vi "FlowCalculation.vi"(6 "order":i32=2, 9 "lowpass":dbl=1.0, 10 "Filter":u16(ring)=2 items=["IIR", "Butterworth", "None"], 11 "X":dbl[](array[numeric]) format="%0.2f") -> (0 "Max amplitude":dbl, 1 "Descending":dbl, 2 "Ascending":dbl, 3 "Flow Graph":T2(graph), 4 "Slopes Out":T1)   [LabVIEW 2013, in "main.lvlib"]
uses:
  main.lvlib
  <vilib>/Analysis/3filter.llb/Filter Passband Type.ctl
  <vilib>/Analysis/3filter.llb/IIR Filter (DBL).vi
  <vilib>/Analysis/3filter.llb/Butterworth Filter (DBL).vi
  <vilib>/Analysis/NI_AALPro.lvlib
  <vilib>/Analysis/NI_AALBase.lvlib
  <vilib>/Analysis/NI_AAL_SigProc.lvlib
panel:
  out "Raw":dbl[](graph)
  out "Derivative Signal":dbl[](graph)
  out "Input Signal":dbl[](graph)
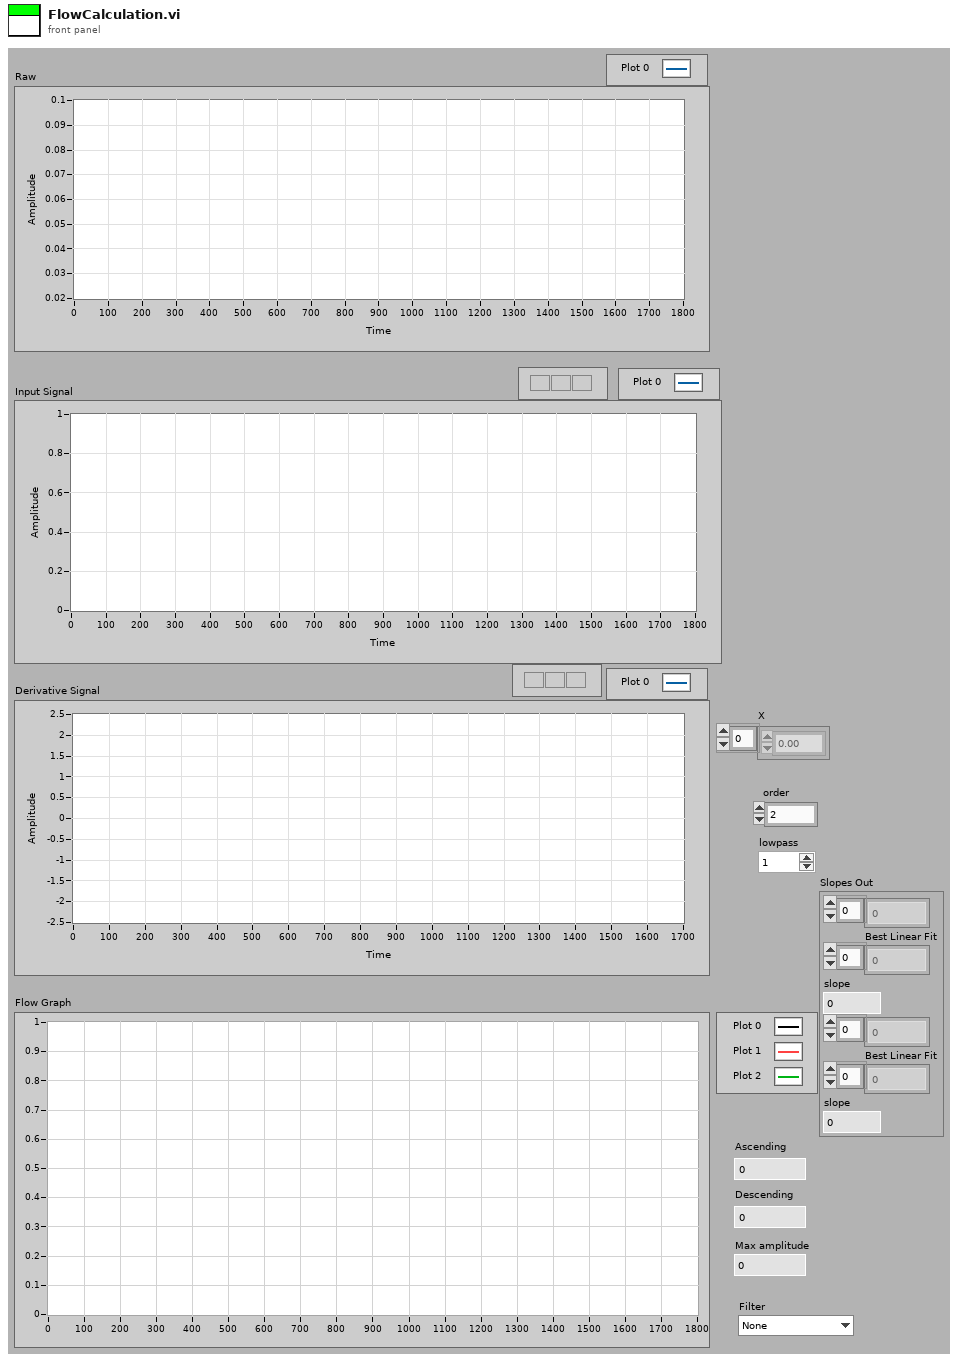
[diagram p1: front panel]
types:
  T1 = cluster{dbl[], "Best Linear Fit":dbl[], "slope":dbl, dbl[], "Best Linear Fit":dbl[], "slope":dbl}
  T2 = cluster{"Array out":dbl[], "Best Linear Fit":dbl[]}[]
  T3 = typedef "NI_AALBase.lvlib/Filter Passband Type.ctl" = enum32{"Lowpass", "Highpass", "Bandpass", "Bandstop"}
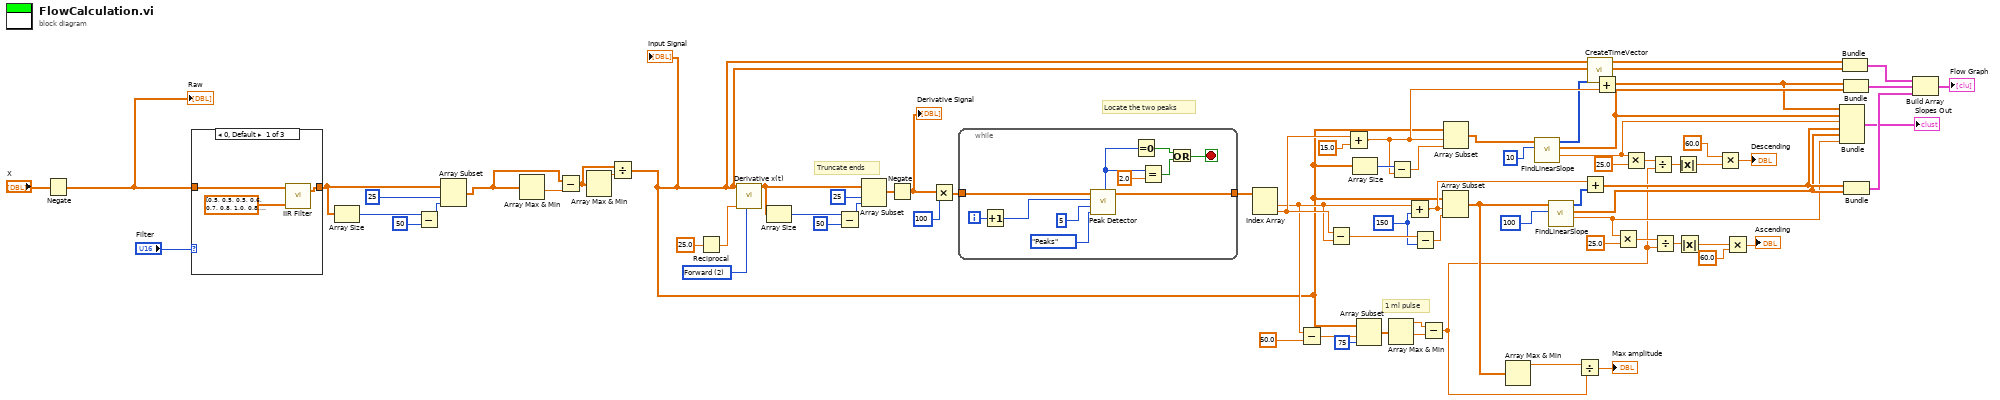
[diagram p0: block diagram]
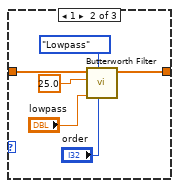
[diagram p2: hidden frame]
diagram:
  w37 = 150
  w75 = u16 2 items=["2nd Order Central", "4th Order Central", "Forward", "Backward"] ("method")
  # "1 ml pulse"
  # "Truncate ends"
  # "Locate the two peaks"
  n1 = Negate(x="X") -> (-x=w19:dbl[])
  "Raw" <- w19
  n2 = case shown="0, Default" "Filter" {
    tunnel: w19 -> [w78 w84 w85]
    tunnel: [w77 w81 w85] -> w12
    frame 0, Default {
      n3 = call-poly <vilib>:"IIR Filter.vi"("Forward Coefficients"=dbl[] [0.5, 0.5, 0.5, 0.6, 0.7, 0.8, 1.0, 0.8, 0.7, 0.6, 0.5, 0.5, 0.5], "X"=w78) -> ("Filtered X"=w77:dbl[])  [unwired: 2 in, 1 out]
    }
    frame 1 {
      n4 = call-poly <vilib>:"Butterworth Filter.vi"("order"="order", "filter type"=Filter_Passband_Type."Lowpass", "low cutoff freq: fl"="lowpass", "sampling freq: fs"=25.0, "X"=w84) -> ("Filtered X"=w81:dbl[])  [unwired: 3 in, 1 out]
    }
    frame 2 {
    }
  }
  n5 = Array Size(array=w12) -> (size(s)=w16:i32)
  n6 = Subtract(x=w16, y=50) -> (x-y=w14:i32)
  n7 = Array Subset(array=w12, index=25, length=w14) -> (w11:dbl[])
  n8 = Array Max & Min(array=w11) -> (min value=w25:dbl)  [unwired: 3 out]
  n9 = Subtract(x=w11, y=w25) -> (x-y=w24:dbl[])
  n10 = Array Max & Min(array=w24) -> (max value=w23:dbl)  [unwired: 3 out]
  n11 = Divide(x=w24, y=w23) -> (x/y=w5:dbl[])
  "Input Signal" <- w5
  n12 = Reciprocal(x=25.0 ("dt")) -> (1/x=w73:dbl)
  n13 = call <vilib>:"Derivative x(t).vi"("method"=w75, "dt"=w73, "X"=w5) -> ("dX/dt"=w72:dbl[])  [unwired: 7 in, 1 out]
  n14 = Array Size(array=w72) -> (size(s)=w71:i32)
  n15 = Subtract(x=w71, y=50) -> (x-y=w69:i32)
  n16 = Array Subset(array=w72, index=25, length=w69) -> (w17:dbl[])
  n17 = Negate(x=w17) -> (-x=w18:dbl[])
  "Derivative Signal" <- w18
  n18 = Multiply(x=w18, y=100) -> (x*y=w22:dbl[])
  n19 = while {
    tunnel: w22 -> [w96]
    tunnel: [w91] -> w26
    i -> [w93]
    stop <- w88 stop-if-true
    n20 = Increment(x=w93) -> (x+1=w92:i32)
    n21 = call <vilib>:"Peak Detector.vi"("peaks/valleys"=enum32{"Peaks", "Valleys"}."Peaks", "width"=5, "threshold"=w92, "X"=w96) -> ("Locations"=w91:dbl[], "# found"=w89:i32)  [unwired: 3 in, 3 out]
    n22 = Equal To 0?(x=w89) -> (x = 0?=w86:bool)
    n23 = Equal?(x=w89, y=2.0) -> (x = y?=w87:bool)
    n24 = Or(x=w86, y=w87) -> (x .or. y?=w88:bool)
  }
  n25 = Index Array(array=w26) -> (element #1=w9:dbl, element #2=w52:dbl)  [unwired: 2 in]
  n26 = Subtract(x=w9, y=50.0) -> (x-y=w7:dbl)
  n27 = Subtract(x=w52, y=w9) -> (x-y=w39:dbl)
  n28 = Add(x=w52, y=15.0) -> (x+y=w61:dbl)
  n29 = Array Size(array=w5) -> (size(s)=w67:i32)
  n30 = Array Subset(array=w5, index=w7, length=75) -> (w4:dbl[])
  n31 = Array Max & Min(array=w4) -> (max value=w3:dbl, min value=w2:dbl)  [unwired: 2 out]
  n32 = Subtract(x=w67, y=w61) -> (x-y=w66:dbl)
  n33 = Add(x=w9, y=w37) -> (x+y=w55:dbl)
  n34 = Subtract(x=w39, y=w37) -> (x-y=w38:dbl)
  n35 = Subtract(x=w3, y=w2) -> (x-y=w1:dbl)
  n36 = Array Subset(array=w5, index=w55, length=w38) -> (w40:dbl[])
  n37 = Array Subset(array=w5, index=w61, length=w66) -> (w64:dbl[])
  n38 = Array Max & Min(array=w40) -> (max value=w10:dbl)  [unwired: 3 out]
  n39 = call "FindLinearSlope.vi"("length"=10, "Array"=w64) -> ("slope"=w32:dbl, "Best Linear Fit"=w33:dbl[], "Array out"=w34:i32[])  [unwired: 7 in]
  n40 = call "FindLinearSlope.vi"("length"=100, "Array"=w40) -> ("slope"=w28:dbl, "Best Linear Fit"=w29:dbl[], "Array out"=w56:i32[])  [unwired: 7 in]
  n41 = Divide(x=w10, y=w1) -> (x/y=→"Max amplitude":dbl)
  n42 = Add(x=w55, y=w56) -> (x+y=w31:dbl[])
  n43 = call "CreateTimeVector.vi"("Array in"=w5) -> ("Array out"=w62:dbl[])  [unwired: 10 in]
  n44 = Add(x=w34, y=w61) -> (x+y=w30:dbl[])
  n45 = Multiply(x=w28, y=25.0) -> (x*y=w51:dbl)
  n46 = Multiply(x=w32, y=25.0) -> (x*y=w49:dbl)
  n47 = Divide(x=w49, y=w1) -> (x/y=w48:dbl)
  n48 = Divide(x=w51, y=w1) -> (x/y=w47:dbl)
  n49 = Absolute Value(x=w48) -> (abs(x)=w43:dbl)
  n50 = Absolute Value(x=w47) -> (abs(x)=w46:dbl)
  n51 = Multiply(x=60.0 ("y"), y=w43) -> (x*y=→"Descending":dbl)
  n52 = Multiply(x=w46, y=60.0) -> (x*y=→"Ascending":dbl)
  n53 = Bundle(w30, "Best Linear Fit"=w33, "slope"=w32, w31, "Best Linear Fit"=w29, "slope"=w28) -> (→"Slopes Out":T1)  [unwired: 1 in]
  n54 = Bundle("Array out"=w62, w5) -> (w60:cluster{"Array out":dbl[], dbl[]})  [unwired: 1 in]
  n55 = Bundle(w30, "Best Linear Fit"=w33) -> (w59:cluster{dbl[], "Best Linear Fit":dbl[]})  [unwired: 1 in]
  n56 = Bundle(w31, "Best Linear Fit"=w29) -> (w35:cluster{dbl[], "Best Linear Fit":dbl[]})  [unwired: 1 in]
  n57 = Build Array(w60, w59, w35) -> (→"Flow Graph":T2)
